vi "DUCOM LAB TEST.vi"() -> ()   [LabVIEW 2021]
panel:
  in  "Home Button 2":bool
  out "error out":errorcluster
  in  "error in (no error)":errorcluster
  in  "Stop Button":bool
  in  "TAB CONTROL":T1(tab)
  in  "SELECT USER":string(combo)
  in  "ABOUT":bool
  in  "CONFRIGURATIONS":bool
  in  "REMOVE USER":bool
  in  "CHANGE PASSWORD":bool
  in  "CREATE NEW USER":bool
  in  "START NEW TEST":bool
  in  "EXIT":bool
  in  "LOGIN":bool
  in  "PASSWORD":string
  out "USER NAME":string
  in  "Home Button":bool
  out "current time":timestamp format="%<%I:%M:%S%2u %p\n%d/%m/%Y>T"
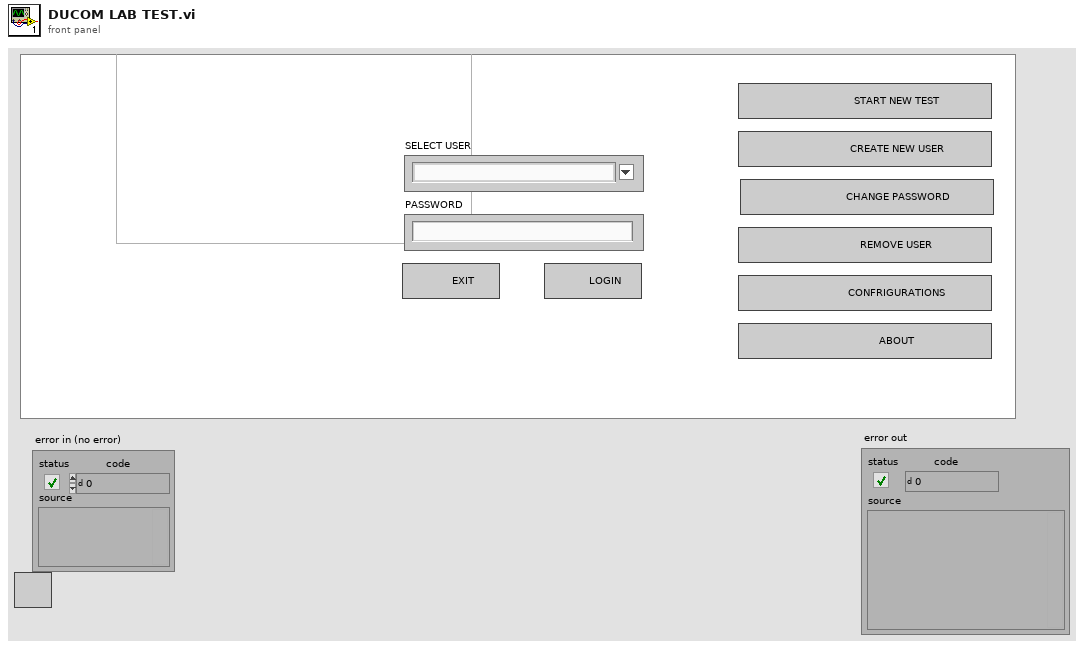
[diagram p1: front panel]
types:
  T1 = enum32{"LOGIN", "ACQUIRE", "CONFRIGURATIONS", "ABOUT"}
  T2 = enum8{"Enabled", "Disabled", "Disabled and Grayed Out"}
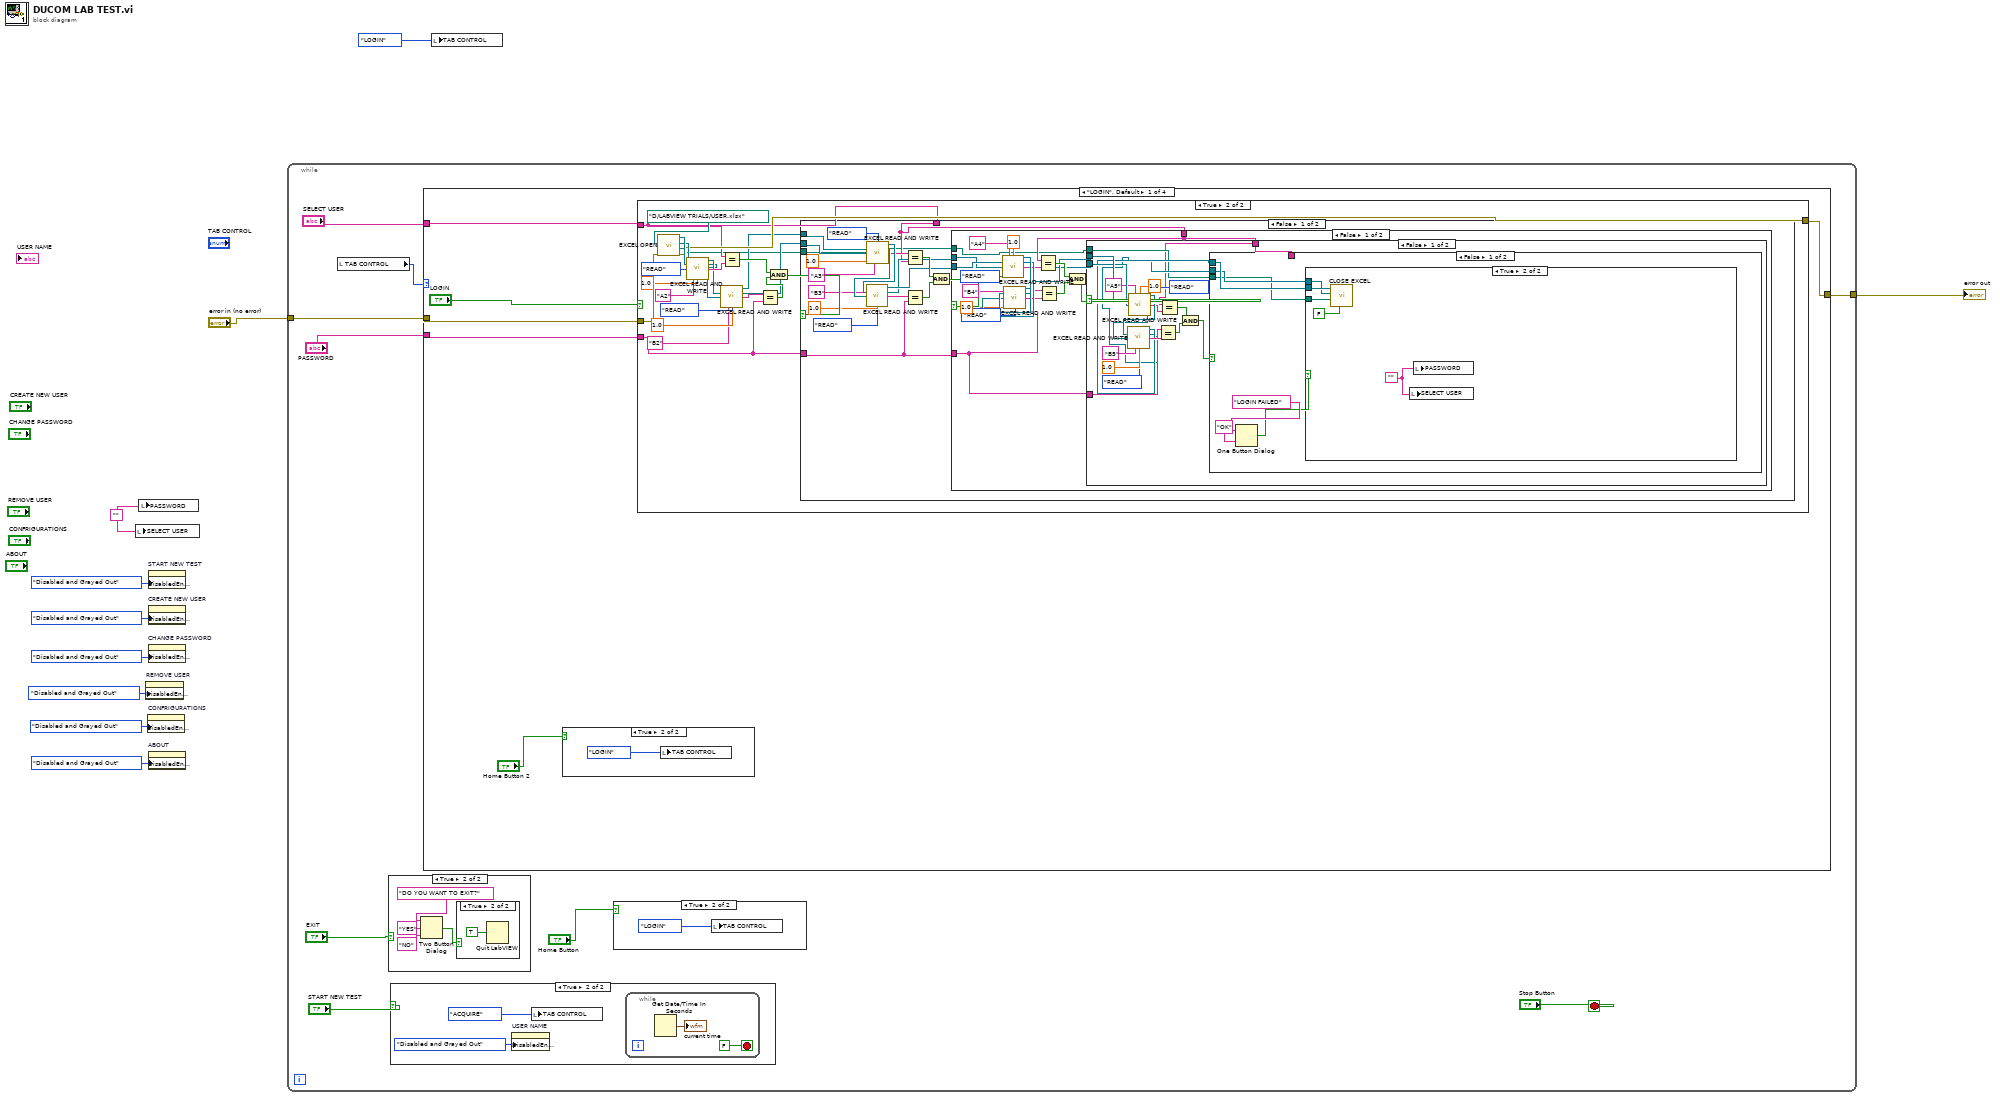
[diagram p0: block diagram]
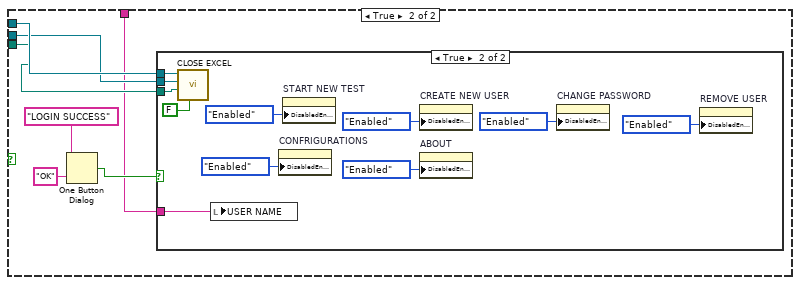
[diagram p9: hidden frame]
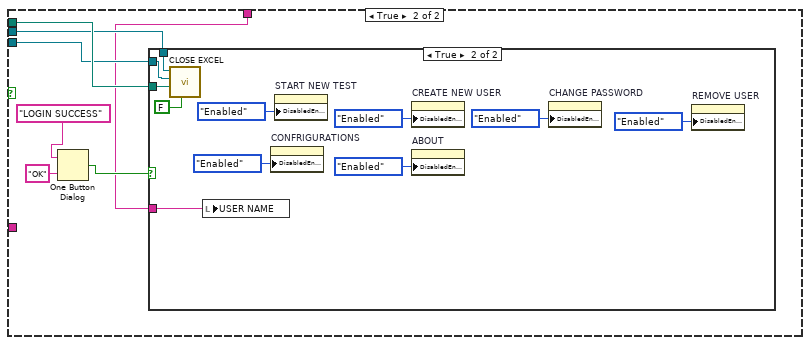
[diagram p11: hidden frame]
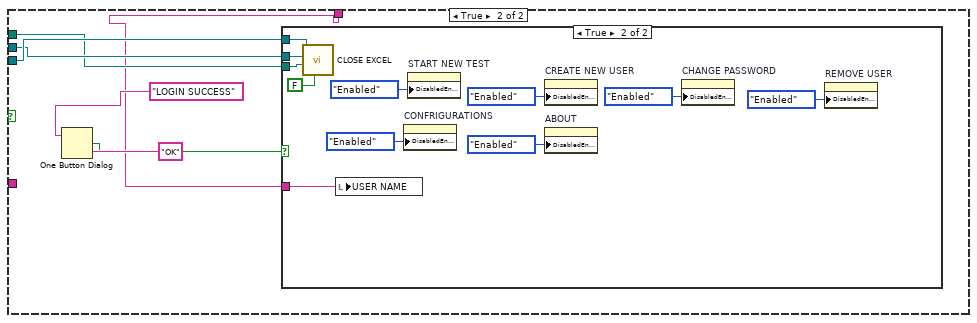
[diagram p13: hidden frame]
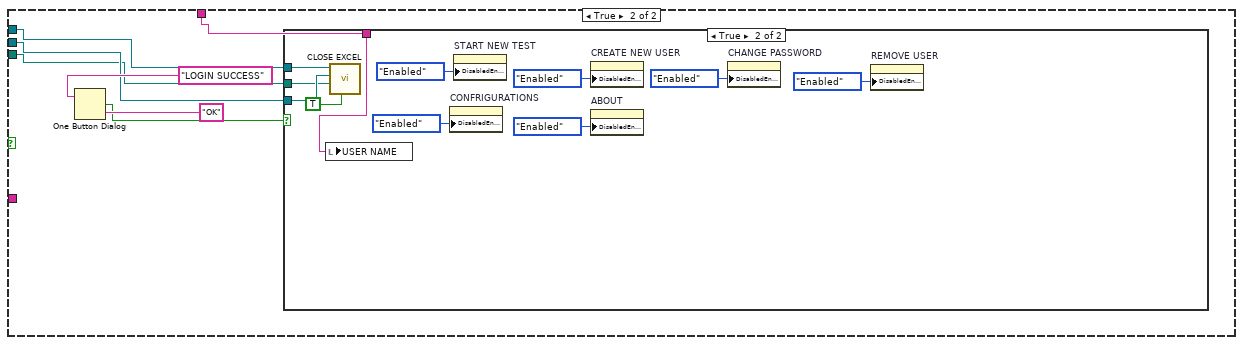
[diagram p15: hidden frame]
diagram:
  w7 = ""
  n1 = local write "SELECT USER"(w7) -> ()
  n2 = local write "PASSWORD"(w7) -> ()
  n3 = property on="REMOVE USER" class="Bool"("DisabledEnum"=T2."Disabled and Grayed Out" ("Disabled")) -> ()  [unwired: 2 in, 2 out]
  n4 = property on="CONFRIGURATIONS" class="Bool"("DisabledEnum"=T2."Disabled and Grayed Out" ("Disabled")) -> ()  [unwired: 2 in, 2 out]
  n5 = property on="START NEW TEST" class="Bool"("DisabledEnum"=T2."Disabled and Grayed Out" ("Disabled")) -> ()  [unwired: 2 in, 2 out]
  n6 = property on="CREATE NEW USER" class="Bool"("DisabledEnum"=T2."Disabled and Grayed Out" ("Disabled")) -> ()  [unwired: 2 in, 2 out]
  n7 = property on="CHANGE PASSWORD" class="Bool"("DisabledEnum"=T2."Disabled and Grayed Out" ("Disabled")) -> ()  [unwired: 2 in, 2 out]
  n8 = property on="ABOUT" class="Bool"("DisabledEnum"=T2."Disabled and Grayed Out" ("Disabled")) -> ()  [unwired: 2 in, 2 out]
  n9 = while {
    tunnel: "error in (no error)" -> [w16]
    tunnel: [w15] -> w9
    stop <- "Stop Button" stop-if-true
    n10 = local read "TAB CONTROL"() -> (w13:T1)
    n11 = case shown="True" "EXIT" {
      frame False {
      }
      frame True {
        n12 = Two Button Dialog(message="DO YOU WANT TO EXIT?", 1:"NO", 2:"YES") -> (T button?=w25:bool)
        n13 = case shown="True" w25 {
          frame False {
          }
          frame True {
            n14 = Quit LabVIEW(quit? (T)=TRUE) -> ()
          }
        }
      }
    }
    n15 = case shown="True" "START NEW TEST" {
      frame False {
      }
      frame True {
        n16 = property on="USER NAME" class="Str"("DisabledEnum"=T2."Disabled and Grayed Out" ("Disabled")) -> ()  [unwired: 2 in, 2 out]
        n17 = local write "TAB CONTROL"(enum32{"LOGIN", "ACQUIRE"}."ACQUIRE" ("TAB CONTROL")) -> ()
        n18 = while {
          stop <- FALSE stop-if-true
          n19 = Get Date/Time In Seconds() -> (seconds since 1Jan1904=→"current time":timestamp)
        }
      }
    }
    n20 = case shown="\"LOGIN\", Default" w13 {
      tunnel: "SELECT USER" -> [w34 _ _ _]
      tunnel: "PASSWORD" -> [w33 _ _ _]
      tunnel: w16 -> [w32 w204 w205 w206]
      tunnel: [w31 w204 w205 w206] -> w15
      frame "LOGIN", Default {
        n21 = case shown="True" "Home Button 2" {
          frame False {
          }
          frame True {
            n22 = local write "TAB CONTROL"(enum32{"LOGIN", "ACQUIRE"}."LOGIN" ("TAB CONTROL")) -> ()
          }
        }
        n23 = case shown="True" "LOGIN" {
          tunnel: w34 -> [_ w39]
          tunnel: w33 -> [_ w40]
          tunnel: w32 -> [w37 w59]
          tunnel: [w37 w43] -> w31
          frame False {
          }
          frame True {
            n24 = call "EXCEL OPEN.vi"("error in (no error)"=w59, "PATH IN"=path "D:/LABVIEW TRIALS/USER.xlsx") -> ("error out"=w43:errorcluster, "PATH OUT"=w38:path, "WORKBOOK OUT"=w57:refnum<k7>, "Excel Application ref  out"=w58:refnum<k7>)  [unwired: 5 in, 1 out]
            n25 = call "EXCEL READ AND WRITE.vi"("CELL"="A2", "SHEET INDEX"=1.0, "Excel.Application REF in"=w58, "Excel._Workbook"=w57, "OPERATION"=enum16{"READ", "WRITE"}."READ") -> ("Excel Application ref out"=w52:refnum<k7>, "WORKBOOK REF OUT"=w51:refnum<k7>, "READING FROM EXCEL"=w53:string)  [unwired: 8 in]
            n26 = call "EXCEL READ AND WRITE.vi"("CELL"="B2", "SHEET INDEX"=1.0, "Excel.Application REF in"=w52, "Excel._Workbook"=w51, "OPERATION"=enum16{"READ", "WRITE"}."READ") -> ("Excel Application ref out"=w42:refnum<k7>, "WORKBOOK REF OUT"=w41:refnum<k7>, "READING FROM EXCEL"=w47:string)  [unwired: 8 in]
            n27 = Equal?(x=w39, y=w53) -> (x = y?=w45:bool)
            n28 = Equal?(x=w47, y=w40) -> (x = y?=w46:bool)
            n29 = And(x=w45, y=w46) -> (x .and. y?=w44:bool)
            n30 = case shown="False" w44 {
              tunnel: w42 -> [w80 w189]
              tunnel: w41 -> [w79 w188]
              tunnel: w40 -> [w62 _]
              tunnel: w39 -> [w63 w186]
              tunnel: w38 -> [w61 w187]
              frame False {
                n31 = call "EXCEL READ AND WRITE.vi"("CELL"="A3", "SHEET INDEX"=1.0, "Excel.Application REF in"=w80, "Excel._Workbook"=w79, "OPERATION"=enum16{"READ", "WRITE"}."READ") -> ("Excel Application ref out"=w75:refnum<k7>, "WORKBOOK REF OUT"=w74:refnum<k7>, "READING FROM EXCEL"=w69:string)  [unwired: 8 in]
                n32 = call "EXCEL READ AND WRITE.vi"("CELL"="B3", "SHEET INDEX"=1.0, "Excel.Application REF in"=w75, "Excel._Workbook"=w74, "OPERATION"=enum16{"READ", "WRITE"}."READ") -> ("Excel Application ref out"=w65:refnum<k7>, "WORKBOOK REF OUT"=w64:refnum<k7>, "READING FROM EXCEL"=w70:string)  [unwired: 8 in]
                n33 = Equal?(x=w69, y=w63) -> (x = y?=w67:bool)
                n34 = Equal?(x=w70, y=w62) -> (x = y?=w68:bool)
                n35 = And(x=w67, y=w68) -> (x .and. y?=w66:bool)
                n36 = case shown="False" w66 {
                  tunnel: w65 -> [w100 w171]
                  tunnel: w64 -> [w99 w170]
                  tunnel: w63 -> [w82 w168]
                  tunnel: w62 -> [w83 _]
                  tunnel: w61 -> [w81 w169]
                  frame False {
                    n37 = call "EXCEL READ AND WRITE.vi"("CELL"="A4", "SHEET INDEX"=1.0, "Excel.Application REF in"=w100, "Excel._Workbook"=w99, "OPERATION"=enum16{"READ", "WRITE"}."READ") -> ("Excel Application ref out"=w95:refnum<k7>, "WORKBOOK REF OUT"=w94:refnum<k7>, "READING FROM EXCEL"=w90:string)  [unwired: 8 in]
                    n38 = call "EXCEL READ AND WRITE.vi"("CELL"="B4", "SHEET INDEX"=1.0, "Excel.Application REF in"=w95, "Excel._Workbook"=w94, "OPERATION"=enum16{"READ", "WRITE"}."READ") -> ("Excel Application ref out"=w85:refnum<k7>, "WORKBOOK REF OUT"=w84:refnum<k7>, "READING FROM EXCEL"=w89:string)  [unwired: 8 in]
                    n39 = Equal?(x=w82, y=w90) -> (x = y?=w87:bool)
                    n40 = Equal?(x=w83, y=w89) -> (x = y?=w88:bool)
                    n41 = And(x=w87, y=w88) -> (x .and. y?=w86:bool)
                    n42 = case shown="False" w86 {
                      tunnel: w85 -> [w120 w151]
                      tunnel: w84 -> [w119 w152]
                      tunnel: w83 -> [w108 _]
                      tunnel: w82 -> [w101 w150]
                      tunnel: w81 -> [w102 w153]
                      frame False {
                        n43 = call "EXCEL READ AND WRITE.vi"("CELL"="A5", "SHEET INDEX"=1.0, "Excel.Application REF in"=w120, "Excel._Workbook"=w119, "OPERATION"=enum16{"READ", "WRITE"}."READ") -> ("Excel Application ref out"=w115:refnum<k7>, "WORKBOOK REF OUT"=w114:refnum<k7>, "READING FROM EXCEL"=w110:string)  [unwired: 8 in]
                        n44 = call "EXCEL READ AND WRITE.vi"("CELL"="B5", "SHEET INDEX"=1.0, "Excel.Application REF in"=w115, "Excel._Workbook"=w114, "OPERATION"=enum16{"READ", "WRITE"}."READ") -> ("Excel Application ref out"=w104:refnum<k7>, "WORKBOOK REF OUT"=w103:refnum<k7>, "READING FROM EXCEL"=w109:string)  [unwired: 8 in]
                        n45 = Equal?(x=w108, y=w109) -> (x = y?=w107:bool)
                        n46 = Equal?(x=w101, y=w110) -> (x = y?=w106:bool)
                        n47 = And(x=w106, y=w107) -> (x .and. y?=w105:bool)
                        n48 = case shown="False" w105 {
                          tunnel: w104 -> [w123 w135]
                          tunnel: w103 -> [w122 w134]
                          tunnel: w102 -> [w121 w133]
                          tunnel: w101 -> [_ w132]
                          frame False {
                            n49 = One Button Dialog(message="LOGIN FAILED", button name ("OK")="OK") -> (true=w124:bool)
                            n50 = case shown="True" w124 {
                              tunnel: w123 -> [_ w131]
                              tunnel: w122 -> [_ w130]
                              tunnel: w121 -> [_ w129]
                              frame False {
                              }
                              frame True {
                                w127 = ""
                                n51 = call "CLOSE EXCEL.vi"("SAVE"=FALSE, "File Path"=w129, "WORKBOOK REF IN"=w130, "APPLICATION REF IN"=w131) -> ()  [unwired: 8 in]
                                n52 = local write "SELECT USER"(w127) -> ()
                                n53 = local write "PASSWORD"(w127) -> ()
                              }
                            }
                          }
                          frame True {
                            n54 = One Button Dialog(message="LOGIN SUCCESS", button name ("OK")="OK") -> (true=w138:bool)
                            n55 = case shown="True" w138 {
                              tunnel: w135 -> [_ w142]
                              tunnel: w134 -> [_ w141]
                              tunnel: w133 -> [_ w140]
                              tunnel: w132 -> [_ w139]
                              frame False {
                              }
                              frame True {
                                n56 = call "CLOSE EXCEL.vi"("SAVE"=FALSE, "File Path"=w140, "WORKBOOK REF IN"=w141, "APPLICATION REF IN"=w142) -> ()  [unwired: 8 in]
                                n57 = local write "USER NAME"(w139) -> ()
                                n58 = property on="CONFRIGURATIONS" class="Bool"("DisabledEnum"=T2."Enabled" ("Disabled")) -> ()  [unwired: 2 in, 2 out]
                                n59 = property on="START NEW TEST" class="Bool"("DisabledEnum"=T2."Enabled" ("Disabled")) -> ()  [unwired: 2 in, 2 out]
                                n60 = property on="CREATE NEW USER" class="Bool"("DisabledEnum"=T2."Enabled" ("Disabled")) -> ()  [unwired: 2 in, 2 out]
                                n61 = property on="ABOUT" class="Bool"("DisabledEnum"=T2."Enabled" ("Disabled")) -> ()  [unwired: 2 in, 2 out]
                                n62 = property on="CHANGE PASSWORD" class="Bool"("DisabledEnum"=T2."Enabled" ("Disabled")) -> ()  [unwired: 2 in, 2 out]
                                n63 = property on="REMOVE USER" class="Bool"("DisabledEnum"=T2."Enabled" ("Disabled")) -> ()  [unwired: 2 in, 2 out]
                              }
                            }
                          }
                        }
                      }
                      frame True {
                        n64 = One Button Dialog(message="LOGIN SUCCESS", button name ("OK")="OK") -> (true=w156:bool)
                        n65 = case shown="True" w156 {
                          tunnel: w153 -> [_ w160]
                          tunnel: w152 -> [_ w159]
                          tunnel: w151 -> [_ w158]
                          tunnel: w150 -> [_ w157]
                          frame False {
                          }
                          frame True {
                            n66 = call "CLOSE EXCEL.vi"("SAVE"=FALSE, "File Path"=w160, "WORKBOOK REF IN"=w159, "APPLICATION REF IN"=w158) -> ()  [unwired: 8 in]
                            n67 = local write "USER NAME"(w157) -> ()
                            n68 = property on="CONFRIGURATIONS" class="Bool"("DisabledEnum"=T2."Enabled" ("Disabled")) -> ()  [unwired: 2 in, 2 out]
                            n69 = property on="START NEW TEST" class="Bool"("DisabledEnum"=T2."Enabled" ("Disabled")) -> ()  [unwired: 2 in, 2 out]
                            n70 = property on="CREATE NEW USER" class="Bool"("DisabledEnum"=T2."Enabled" ("Disabled")) -> ()  [unwired: 2 in, 2 out]
                            n71 = property on="ABOUT" class="Bool"("DisabledEnum"=T2."Enabled" ("Disabled")) -> ()  [unwired: 2 in, 2 out]
                            n72 = property on="CHANGE PASSWORD" class="Bool"("DisabledEnum"=T2."Enabled" ("Disabled")) -> ()  [unwired: 2 in, 2 out]
                            n73 = property on="REMOVE USER" class="Bool"("DisabledEnum"=T2."Enabled" ("Disabled")) -> ()  [unwired: 2 in, 2 out]
                          }
                        }
                      }
                    }
                  }
                  frame True {
                    n74 = One Button Dialog(message="LOGIN SUCCESS", button name ("OK")="OK") -> (true=w172:bool)
                    n75 = case shown="True" w172 {
                      tunnel: w171 -> [_ w185]
                      tunnel: w170 -> [_ w184]
                      tunnel: w169 -> [_ w183]
                      tunnel: w168 -> [_ w175]
                      frame False {
                      }
                      frame True {
                        n76 = call "CLOSE EXCEL.vi"("SAVE"=FALSE, "File Path"=w183, "WORKBOOK REF IN"=w184, "APPLICATION REF IN"=w185) -> ()  [unwired: 8 in]
                        n77 = local write "USER NAME"(w175) -> ()
                        n78 = property on="CONFRIGURATIONS" class="Bool"("DisabledEnum"=T2."Enabled" ("Disabled")) -> ()  [unwired: 2 in, 2 out]
                        n79 = property on="START NEW TEST" class="Bool"("DisabledEnum"=T2."Enabled" ("Disabled")) -> ()  [unwired: 2 in, 2 out]
                        n80 = property on="CREATE NEW USER" class="Bool"("DisabledEnum"=T2."Enabled" ("Disabled")) -> ()  [unwired: 2 in, 2 out]
                        n81 = property on="ABOUT" class="Bool"("DisabledEnum"=T2."Enabled" ("Disabled")) -> ()  [unwired: 2 in, 2 out]
                        n82 = property on="CHANGE PASSWORD" class="Bool"("DisabledEnum"=T2."Enabled" ("Disabled")) -> ()  [unwired: 2 in, 2 out]
                        n83 = property on="REMOVE USER" class="Bool"("DisabledEnum"=T2."Enabled" ("Disabled")) -> ()  [unwired: 2 in, 2 out]
                      }
                    }
                  }
                }
              }
              frame True {
                n84 = One Button Dialog(message="LOGIN SUCCESS", button name ("OK")="OK") -> (true=w190:bool)
                n85 = case shown="True" w190 {
                  tunnel: w189 -> [_ w203]
                  tunnel: w188 -> [_ w202]
                  tunnel: w187 -> [_ w201]
                  tunnel: w186 -> [_ w193]
                  frame False {
                  }
                  frame True {
                    n86 = local write "USER NAME"(w193) -> ()
                    n87 = call "CLOSE EXCEL.vi"("SAVE"=TRUE, "File Path"=w201, "WORKBOOK REF IN"=w202, "APPLICATION REF IN"=w203) -> ()  [unwired: 8 in]
                    n88 = property on="CONFRIGURATIONS" class="Bool"("DisabledEnum"=T2."Enabled" ("Disabled")) -> ()  [unwired: 2 in, 2 out]
                    n89 = property on="START NEW TEST" class="Bool"("DisabledEnum"=T2."Enabled" ("Disabled")) -> ()  [unwired: 2 in, 2 out]
                    n90 = property on="CREATE NEW USER" class="Bool"("DisabledEnum"=T2."Enabled" ("Disabled")) -> ()  [unwired: 2 in, 2 out]
                    n91 = property on="ABOUT" class="Bool"("DisabledEnum"=T2."Enabled" ("Disabled")) -> ()  [unwired: 2 in, 2 out]
                    n92 = property on="CHANGE PASSWORD" class="Bool"("DisabledEnum"=T2."Enabled" ("Disabled")) -> ()  [unwired: 2 in, 2 out]
                    n93 = property on="REMOVE USER" class="Bool"("DisabledEnum"=T2."Enabled" ("Disabled")) -> ()  [unwired: 2 in, 2 out]
                  }
                }
              }
            }
          }
        }
      }
      frame "ACQUIRE" {
      }
      frame "CONFRIGURATIONS" {
      }
      frame "ABOUT" {
      }
    }
    n94 = case shown="True" "Home Button" {
      frame False {
      }
      frame True {
        n95 = local write "TAB CONTROL"(enum32{"LOGIN", "ACQUIRE"}."LOGIN" ("TAB CONTROL")) -> ()
      }
    }
  }
  "error out" <- w9
  n96 = local write "TAB CONTROL"(enum32{"LOGIN", "ACQUIRE"}."LOGIN" ("TAB CONTROL")) -> ()
